vi "Que.vi"(4 "error in (no error)":errorcluster caption="에러 입력(에러 없음)", 5 "Que info":T1, 6 "Muticol listbox in":string[][](array[string]), 7 "Data stack IN":refnum<class "Retrieved Data.lvclass">[](array[class])) -> (0 "에러 출력":errorcluster, 2 "Muticol listbox out":string[][](array[string]), 3 "Data stack OUT":refnum<class "Retrieved Data.lvclass">[](array[class]))   [LabVIEW 2017, in "Retrieved Data.lvclass"]
uses:
  Retrieved Data.lvclass
panel:
  in  "Retrieved Data.lvclass":refnum<class "Retrieved Data.lvclass">
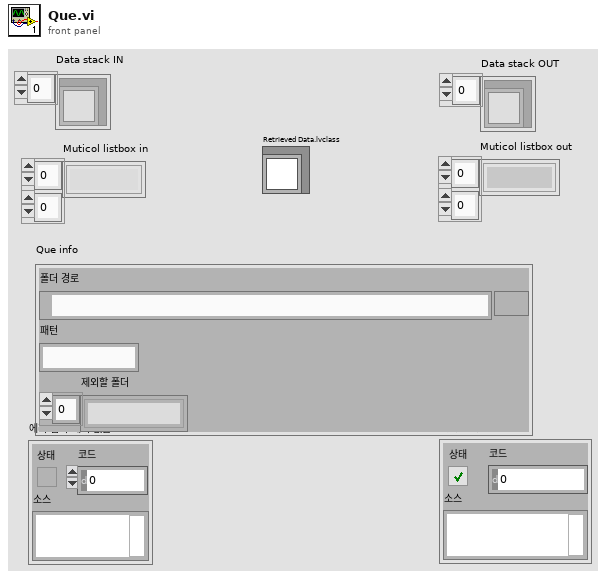
[diagram p1: front panel]
types:
  T1 = cluster{"Folder Path":path, "Que":string, "Folders to Exclude":string[]}
  T2 = cluster{"Selected event":dbl[][], "Interevent interval":dbl[], "Summary":cluster{"Event #":i32, "Amplitude (selected)":dbl, "Frequency":dbl}}
  T3 = cluster{"EVT":dbl[][], "Interevent interval":dbl[], "Summary":cluster{"Event #":i32, "Amplitude (total)":dbl, "Frequency":dbl}}
  T4 = cluster{"Event #":i32, "Amplitude (selected)":dbl, "Frequency":dbl}
  T5 = cluster{"Event #":i32, "Amplitude (total)":dbl, "Frequency":dbl}
  T6 = cluster{"Que":string, string[], string[][], "Input + Mean,SD,SEM":dbl[][], dbl[], dbl[], string[], "원소":string[]}
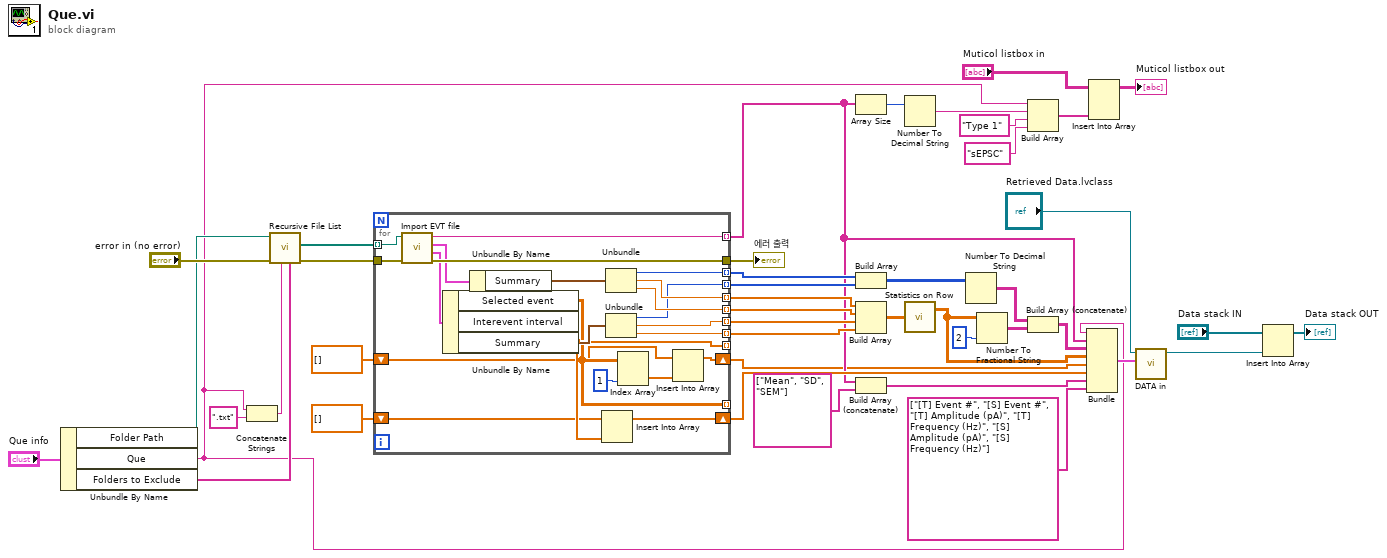
[diagram p0: block diagram]
diagram:
  n1 = Unbundle By Name("Que info") -> ("Folder Path"=w16:path, "Que"=w2:string, "Folders to Exclude"=w15:string[])
  n2 = Concatenate Strings(w2, ".txt" ("문자열")) -> (w1:string)
  n3 = call <vilib>:"Recursive File List.vi"("Folders to Exclude"=w15, "pattern"=w1, "error in (no error)"="error in (no error)", "Folder Path"=w16) -> ("error out"=w42:errorcluster, "All Files in Dir"=w43:path[])  [unwired: 3 in, 3 out]
  n4 = for {
    tunnel: w43 -> [w65] mode=indexing
    tunnel: [w64] -> w25 mode=indexing
    tunnel: w42 -> [w63]
    tunnel: [w62] -> w8
    tunnel: [w59] -> w36 mode=indexing
    tunnel: [w58] -> w41 mode=indexing
    tunnel: [w57] -> w40 mode=indexing
    tunnel: [w54] -> w35 mode=indexing
    tunnel: [w53] -> w38 mode=indexing
    tunnel: [w52] -> w37 mode=indexing
    tunnel: [w48] -> _ mode=indexing
    tunnel: [w51] -> _ mode=indexing
    shift-right: [w50] -> w28
    shift-left: dbl[] [] -> [w49]
    shift-right: [w45] -> w12
    shift-left: dbl[] [] -> [w44]
    n5 = call "Import EVT file.vi"("error in (no error)"=w63, "file path"=w65) -> ("error out"=w62:errorcluster, "Selected"=w56:T2, "Total"=w61:T3, "File name"=w64:string)  [unwired: 2 in]
    n6 = Unbundle By Name(w56) -> ("Selected event"=w48:dbl[][], "Interevent interval"=w51:dbl[], "Summary"=w55:T4)
    n7 = Unbundle By Name(w61) -> ("Summary"=w60:T5)
    n8 = Insert Into Array(array=w49, new element=w51) -> (w50:dbl[])  [unwired: 1 in]
    n9 = Unbundle(w60) -> ("Event #"=w59:i32, "Amplitude (total)"=w58:dbl, "Frequency"=w57:dbl)
    n10 = Unbundle(w55) -> ("Event #"=w54:i32, "Amplitude (selected)"=w53:dbl, "Frequency"=w52:dbl)
    n11 = Index Array(array=w48, index (col)=1 ("비활성화된 인덱스 (열)")) -> (element=w46:dbl[])  [unwired: 1 in]
    n12 = Insert Into Array(array=w44, new element=w46) -> (w45:dbl[])  [unwired: 1 in]
  }
  "에러 출력" <- w8
  n13 = Array Size(array=w25) -> (size(s)=w24:i32)
  n14 = Build Array(w36, w35) -> (w7:i32[][])
  n15 = Build Array(w41, w40, w38, w37) -> (w39:dbl[][])
  n16 = Build Array (concatenate)(w25, string[] ["Mean", "SD", "SEM"] ("원소")) -> (w11:string[])
  n17 = Number To Decimal String(number=w24) -> (decimal integer string=w23:string)  [unwired: 1 in]
  n18 = call <userlib>:"Statistics on Row.vi"("Input"=w39) -> ("Input + Mean,SD,SEM"=w29:dbl[][])  [unwired: 1 out]
  n19 = Number To Decimal String(number=w7) -> (decimal integer string=w6:string[][])  [unwired: 1 in]
  n20 = Number To Fractional String(number=w29, precision (6)=i16 2 ("정밀도(6)")) -> (F-format string=w5:string[][])  [unwired: 2 in]
  n21 = Build Array(w2, w23, "Type 1" ("원소"), "sEPSC" ("원소")) -> (w18:string[])
  n22 = Build Array (concatenate)(w6, w5) -> (w4:string[][])
  n23 = Bundle("Que"=w2, w25, w4, "Input + Mean,SD,SEM"=w29, w12, w28, w11, "원소"=string[] ["[T] Event #", "[S] Event #", "[T] Amplitude (pA)", "[T] Frequency (Hz)", "[S] Amplitude (pA)", "[S] Frequency (Hz)"]) -> (w9:T6)  [unwired: 1 in]
  n24 = Insert Into Array(array="Muticol listbox in", new element=w18) -> (→"Muticol listbox out":string[][])  [unwired: 2 in]
  n25 = call "DATA in.vi"("출력 클러스터"=w9, "Retrieved Data.lvclass"="Retrieved Data.lvclass") -> ("Retrieved Data.lvclass 2"=w14:refnum<class "Retrieved Data.lvclass">)  [unwired: 5 in]
  n26 = Insert Into Array(array="Data stack IN", new element=w14) -> (→"Data stack OUT":refnum<class "Retrieved Data.lvclass">[])  [unwired: 1 in]
